vi "7p1_HW_Task1D_doanbs.vi"() -> ()   [LabVIEW 2016]
uses:
  <vilib>/express/express arith-compare/Formula/XNode/ExpressFormulaBlockNode.xnode
panel:
  out "Units":string
  in  "Units":string(combo)
  out "C":dbl
  out "b":dbl
  in  "A":dbl
  in  "B":dbl
  in  "a":dbl
  in  "c":dbl
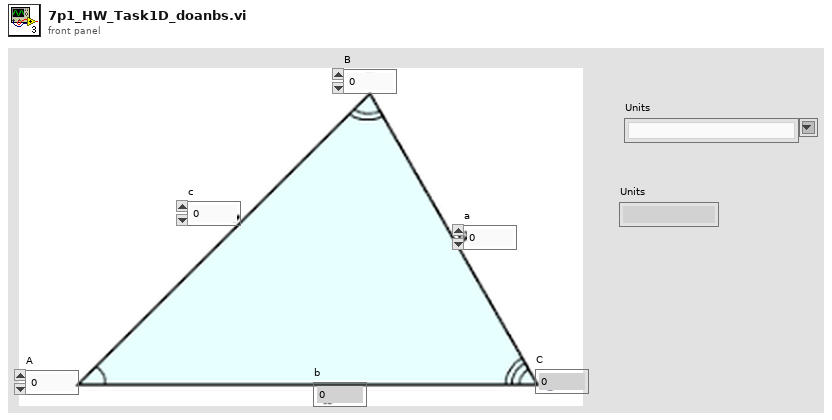
[diagram p1: front panel]
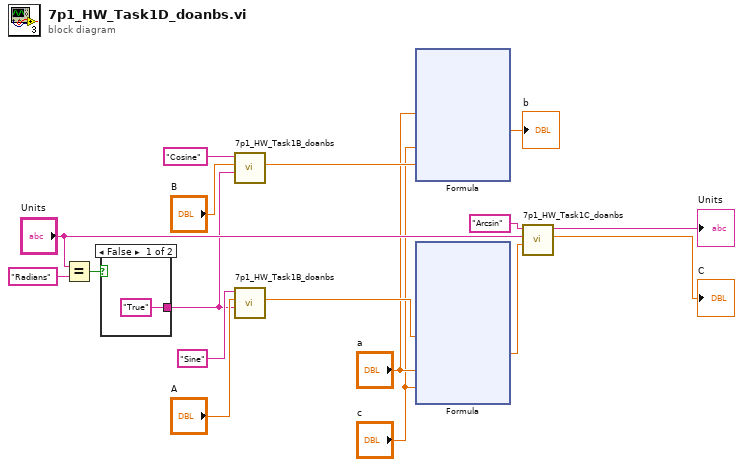
[diagram p0: block diagram]
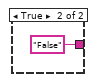
[diagram p2: hidden frame]
diagram:
  n1 = Equal?(x="Units", y="Radians") -> (x = y?=w14:bool)
  n2 = case shown="False" w14 {
    tunnel: ["True" "False"] -> w6
    frame False {
    }
    frame True {
    }
  }
  n3 = call "7p1_HW_Task1B_doanbs.vi"("Convert?"=w6, "th, Theta"="B", "Trig Function"="Cosine") -> ("Calculated Value"=w4:dbl)  [unwired: 7 in, 1 out]
  n4 = call "7p1_HW_Task1B_doanbs.vi"("Convert?"=w6, "th, Theta"="A", "Trig Function"="Sine") -> ("Calculated Value"=w16:dbl)  [unwired: 7 in, 1 out]
  n5 = xnode "Formula"("a"="a", "c"="c", "B"=w4) -> ("Result"=→"b":dbl)  [unwired: 1 in, 1 out]
  n6 = xnode "Formula"("A"=w16, "a"="a", "c"="c") -> ("Result"=w11:dbl)  [unwired: 1 in, 1 out]
  n7 = call "7p1_HW_Task1C_doanbs.vi"("x, Original Value"=w11, "Output in Degrees or Radians?"="Units", "Inverse Trig Function"="Arcsin") -> ("th, Theta"=→"C":dbl, "Units"=→"Units":string)  [unwired: 7 in]
